vi "Fluence in multiple areas.vi"(0 "Analyze Fluence in":refnum<class "Analyze Fluence.lvclass">, 5 "Image in":T1, 7 "Energy":dbl, 9 "Create Overlay(T)?":bool, 11 "error in (no error)":errorcluster) -> (4 "Analyze Fluence out":refnum<class "Analyze Fluence.lvclass">, 6 "Image Dst Out":T1, 8 "Max Fluence J/cm^2":dbl, 10 "fluence infos":T2[](array[typedef]), 15 "error out":errorcluster)   [LabVIEW 2009, in "Analyze.lvlib" / "Analyze Fluence.lvclass"]
uses:
  Analyze Fluence.lvclass
  Fluence Info.ctl
  <vilib>/vision/Image Controls.llb/IMAQ Image.ctl
  Analyze Fluence.lvclass/Analyze Fluence.ctl
  <vilib>/vision/NI_Vision_Development_Module.lvlib
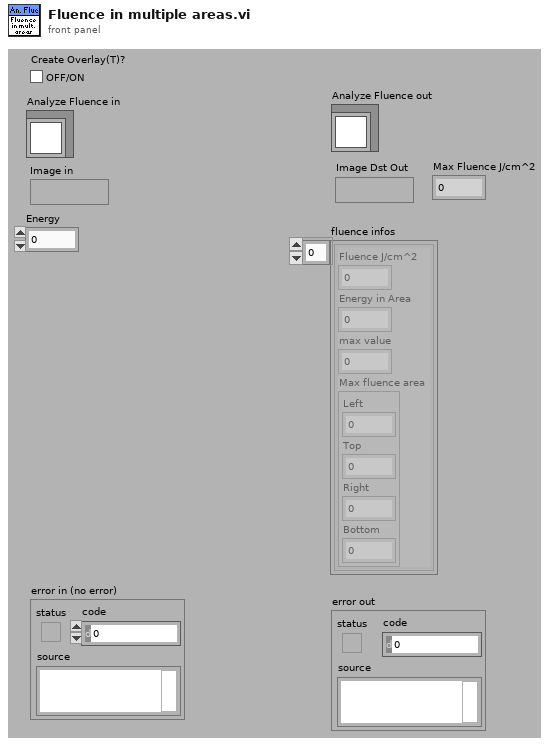
[diagram p1: front panel]
types:
  T1 = typedef "IMAQ Image.ctl" = refnum<image>
  T2 = typedef "Analyze.lvlib/Analyze Fluence.lvclass/Fluence Info.ctl" = cluster{"Fluence J/cm^2":dbl, "Energy in Area":dbl, "max value":i64, "Max fluence area":cluster{"Left":i32, "Top":i32, "Right":i32, "Bottom":i32}}
  T3 = typedef "ROI Descriptor" = cluster{"Global Rectangle":i32[], "Contours":cluster{"ID":enum32{"External", "Internal"}, "Type":u32, "Coordinates":i32[]}[]}
  T4 = typedef "IMAQ Rectangle" = cluster{"Left":i32, "Top":i32, "Right":i32, "Bottom":i32, "Rotation":dbl}
  T5 = typedef "Image Type" = u32
  T6 = cluster{"Left":i32, "Top":i32, "Right":i32, "Bottom":i32}
  T7 = cluster{"Fluence J/cm^2":dbl, "Energy in Area":dbl, "max value":i64, "Max fluence area":cluster{"Left":i32, "Top":i32, "Right":i32, "Bottom":i32}}
  T8 = cluster{"Desired Font (Application)":enum16{"User-specified Font", "Application Font", "System Font", "Dialog Font"}, "[User-specified Font]":cluster{"Font Name":string, "Size":i16, "Strikeout?":bool, "Italic?":bool, "Underline?":bool, "Outline?":bool, "Shadow?":bool, "Bold?":bool, "Rotation Angle":dbl}, "Horizontal Alignment":i16, "Vertical Alignment":i16}
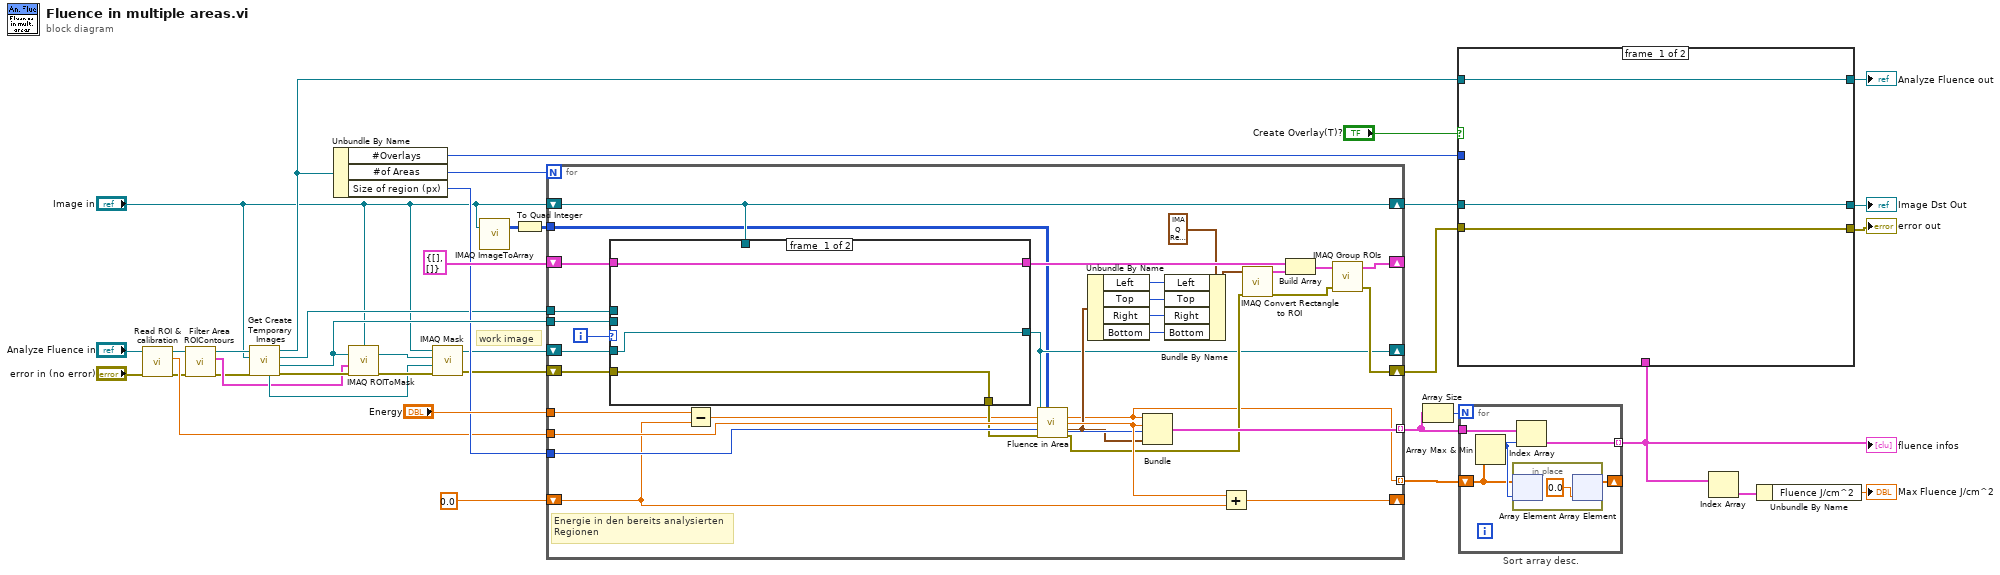
[diagram p0: block diagram]
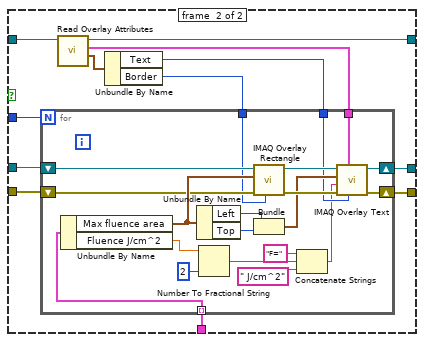
[diagram p2: hidden frame]
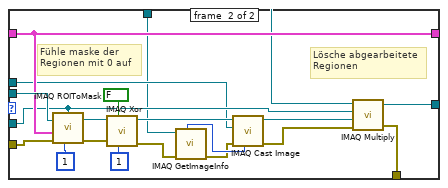
[diagram p3: hidden frame]
diagram:
  # "work image"
  n1 = call-dynamic "Read ROI & calibration.vi"("error in (no error)"="error in (no error)", "Analyze BaseClass in"="Analyze Fluence in") -> ("error out"=w8:errorcluster, "calibration mm/px"=w14:dbl, "Analyze BaseClass out"=w12:refnum<class "Analyze Fluence.lvclass">)  [unwired: 6 in, 1 out]
  n2 = call-dynamic "Filter Area ROIContours.vi"("error in (no error)"=w8, "Analyze BaseClass in"=w12) -> ("error out"=w7:errorcluster, "ROI of Area type"=w13:T3, "Analyze BaseClass out"=w10:refnum<class "Analyze Fluence.lvclass">)  [unwired: 7 in]
  n3 = call-dynamic "Get Create Temporary Images.vi"("error in (no error)"=w7, "Image in"="Image in", "Analyze BaseClass in"=w10) -> ("error out"=w20:errorcluster, "image mask"=w22:T1, "work image"=w4:T1, "Analyze BaseClass out"=w15:refnum<class "Analyze Fluence.lvclass">, "masked image"=w21:T1)  [unwired: 4 in]
  n4 = Unbundle By Name(w15) -> ("#Overlays"=w25:i32, "#of Areas"=w26:i32, "Size of region (px)"=w17:i32)
  n5 = call "IMAQ ROIToMask"("error in (no error)"=w20, "ROI Descriptor"=w13, "Image"=w22, "Image Model"="Image in") -> ("error out"=w24:errorcluster, "Image Out"=w36:T1)  [unwired: 2 in, 1 out]
  n6 = call "IMAQ Mask"("error in (no error)"=w24, "Image Dst"=w21, "Image Mask"=w36, "Image Src"="Image in") -> ("error out"=w5:errorcluster, "Image Dst Out"=w6:T1)  [unwired: 1 in]
  n7 = call "IMAQ ImageToArray"("Image"="Image in") -> ("Image Pixels (I16)"=w3:i16[][])  [unwired: 3 in, 4 out]
  n8 = To Quad Integer(1:w3) -> (0:w1:i64[][])
  n9 = for {
    N: w26 -> [_]
    tunnel: "Energy" -> [w72]
    tunnel: w14 -> [w71]
    tunnel: w17 -> [w70]
    shift-right: [w69] -> _
    shift-left: T3 {"Global Rectangle"=[], "Contours"=[]} ("ROI Descriptor 2") -> [w63]
    tunnel: w22 -> [w68]
    tunnel: w4 -> [w66]
    shift-right: [w42] -> _
    shift-left: w6 -> [w43]
    shift-right: [w46] -> w29
    shift-left: w5 -> [w67]
    shift-right: [w65] -> _
    shift-left: 0.0 ("Energy in Area") -> [w64]
    tunnel: [w44] -> w18 mode=indexing
    shift-right: [w40] -> w31
    shift-left: "Image in" -> [w40]
    tunnel: [w47] -> w19 mode=indexing
    tunnel: w1 -> [w39]
    i -> [w50]
    # "Energie in den bereits analysierten \nRegionen"
    n10 = case shown="1, Default" w50 {
      tunnel: w68 -> [_ w90]
      tunnel: w67 -> [w75 w89]
      tunnel: w66 -> [_ w77]
      tunnel: w43 -> [w74 w78]
      tunnel: w63 -> [w73 w82]
      tunnel: [w75 w92] -> w55
      tunnel: [w74 w91] -> w42
      tunnel: [w73 w82] -> w48
      tunnel: w40 -> [_ w76]
      frame #0 {
      }
      frame #1 {
        # "Lösche abgearbeitete\nRegionen"
        # "Fühle maske der\nRegionen mit 0 auf"
        n11 = call "IMAQ ROIToMask"("error in (no error)"=w89, "ROI Descriptor"=w82, "Filling Value (255)"=1 ("Background Value (0)"), "Image"=w90, "Image Model"=w78) -> ("error out"=w85:errorcluster, "Image Out"=w84:T1)  [unwired: 1 in, 1 out]
        n12 = call "IMAQ Xor"("Constant"=1, "Xor/Xnor (Xor)"=FALSE ("And/Nand (And)"), "error in (no error)"=w85, "Image Src A"=w84) -> ("error out"=w80:errorcluster, "Image Dst Out"=w83:T1)  [unwired: 6 in]
        n13 = call "IMAQ GetImageInfo"("error in (no error)"=w80, "Image"=w76) -> ("error out"=w79:errorcluster, "Image Type"=w81:T5)  [unwired: 2 in, 6 out]
        n14 = call "IMAQ Cast Image"("Image Type"=w81, "error in (no error)"=w79, "Image Dst"=w77, "Image Src"=w83) -> ("error out"=w93:errorcluster, "Image Dst Out"=w94:T1)  [unwired: 6 in]
        n15 = call "IMAQ Multiply"("Image Src A"=w76, "Image Dst"=w78, "Image Src B"=w94, "error in (no error)"=w93) -> ("Image Dst Out"=w91:T1, "error out"=w92:errorcluster)  [unwired: 3 in]
      }
    }
    n16 = Subtract(x=w72, y=w64) -> (x-y=w54:dbl)
    n17 = call "Fluence in Area.vi"("Masked Image"=w42, "Origin Image"=w39, "Energie"=w54, "calibration mm/px"=w71, "Size of region"=w70, "error in (no error)"=w55) -> ("Fluence J/cm^2"=w44:dbl, "Energy in Area"=w53:dbl, "Max fluence area"=w51:T6, "max value"=w52:i64, "error out"=w45:errorcluster)  [unwired: 5 in]
    n18 = Unbundle By Name(w51) -> ("Left"=w59:i32, "Top"=w60:i32, "Right"=w61:i32, "Bottom"=w62:i32)
    n19 = Bundle("Fluence J/cm^2"=w44, "Energy in Area"=w53, "max value"=w52, "Max fluence area"=w51) -> (w47:T7)  [unwired: 1 in]
    n20 = Bundle By Name(cluster=T4 {"Left"=0, "Top"=0, "Right"=0, "Bottom"=0, "Rotation"=0.0} ("Rectangle"), "Left"=w59, "Top"=w60, "Right"=w61, "Bottom"=w62) -> (w58:T4)
    n21 = Add(x=w53, y=w64) -> (x+y=w65:dbl)
    n22 = call "IMAQ Convert Rectangle to ROI"("error in (no error)"=w45, "Rectangle"=w58) -> ("error out"=w49:errorcluster, "ROI Descriptor"=w57:T3)  [unwired: 7 in]
    n23 = Build Array(w48, w57) -> (w56:T3[])
    n24 = call "IMAQ Group ROIs"("error in (no error)"=w49, "ROI Descriptors"=w56) -> ("error out"=w46:errorcluster, "ROI Descriptor out"=w69:T3)  [unwired: 2 in]
  }
  n25 = Array Size(array=w19) -> (size(s)=w27:i32)
  n26 = for "Sort array desc." {
    N: w27 -> [_]
    shift-right: [w95] -> _
    shift-left: w18 -> [w96]
    tunnel: w19 -> [w99]
    tunnel: [w98] -> w32 mode=indexing
    n27 = Array Max & Min(array=w96) -> (max index (indices)=w97:i32)  [unwired: 3 out]
    n28 = in-place {
      n29 = in-place-array #1(w96, w97) -> ()  [unwired: 1 out]
      n30 = in-place-array #1(0.0 ("element")) -> (w95:dbl[])  [unwired: 1 out]
    }
    n31 = Index Array(array=w99, index=w97) -> (element=w98:T7)
  }
  "fluence infos" <- w32
  n32 = case shown="True" "Create Overlay(T)?" {
    tunnel: w32 -> [_ w115]
    tunnel: w31 -> [w103 w114]
    tunnel: [w103 w113] -> w30
    tunnel: w29 -> [w102 w112]
    tunnel: [w102 w111] -> w28
    tunnel: w25 -> [_ w108]
    tunnel: [w101 w107] -> w16
    tunnel: w15 -> [w101 w106]
    frame #0 {
    }
    frame #1 {
      n33 = call-dynamic "Read Overlay Attributes.vi"("Analyze BaseClass in"=w106) -> ("Overlay colors"=w105:cluster{"Border":u32, "Text":u32}, "Font, Size & Style"=w104:T8, "Analyze BaseClass out"=w107:refnum<class "Analyze Fluence.lvclass">)  [unwired: 7 in, 1 out]
      n34 = Unbundle By Name(w105) -> ("Text"=w110:u32, "Border"=w109:u32)
      n35 = for {
        N: w108 -> [_]
        tunnel: w115 -> [w135] mode=indexing
        shift-right: [w124] -> w113
        shift-left: w114 -> [w125]
        shift-right: [w123] -> w111
        shift-left: w112 -> [w122]
        tunnel: w110 -> [w121]
        tunnel: w109 -> [w120]
        tunnel: w104 -> [w119]
        n36 = Unbundle By Name(w135) -> ("Max fluence area"=w127:T6, "Fluence J/cm^2"=w126:dbl)
        n37 = Unbundle By Name(w127) -> ("Left"=w128:i32, "Top"=w129:i32)
        n38 = Number To Fractional String(number=w126, precision (6)=i16 2) -> (F-format string=w132:string)  [unwired: 2 in]
        n39 = call "IMAQ Overlay Rectangle"("Color"=w120, "error in (no error)"=w122, "Rectangle"=w127, "Image"=w125) -> ("error out"=w134:errorcluster, "Image Out"=w133:T1)  [unwired: 6 in]
        n40 = Bundle("Left"=w128, "Top"=w129) -> (w130:cluster{"Left":i32, "Top":i32})  [unwired: 1 in]
        n41 = Concatenate Strings("F=" ("string"), w132, " J/cm^2" ("string")) -> (w118:string)
        n42 = call "IMAQ Overlay Text"("Text Color (black)"=w121, "Font, Size & Style"=w119, "error in (no error)"=w134, "String"=w118, "Origin"=w130, "Image"=w133) -> ("error out"=w123:errorcluster, "Image Out"=w124:T1)  [unwired: 4 in]
      }
    }
  }
  "error out" <- w28
  "Image Dst Out" <- w30
  "Analyze Fluence out" <- w16
  n43 = Index Array(array=w32) -> (element=w34:T7)  [unwired: 1 in]
  n44 = Unbundle By Name(w34) -> ("Fluence J/cm^2"=→"Max Fluence J/cm^2":dbl)
